vi "IMAQdx Read Memory2.vi"(8 "error in":errorcluster, 9 "Memory Size":u32, 10 "Offset":u64=4042262528 format="%.0x", 11 "Session In":T1) -> (0 "error out":errorcluster, 1 "Value":string, 3 "Session Out":T1)   [LabVIEW 2020, in "NI_Vision_Acquisition_Software.lvlib"]
doc: "Accesses registers on the camera and reads a string from the camera."
uses:
  NI_Vision_Acquisition_Software.lvlib
  IMAQdx.ctl
  niimaqdx.dll
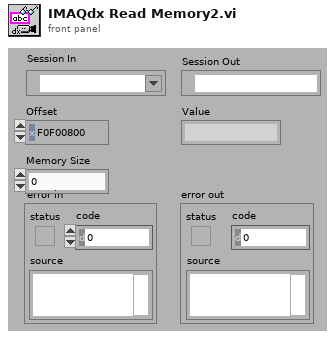
[diagram p1: front panel]
types:
  T1 = typedef "IMAQdx.ctl" = refnum<k21>
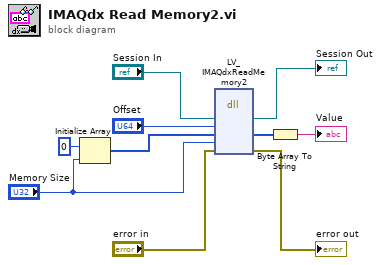
[diagram p0: block diagram]
diagram:
  n1 = Initialize Array(u8 0 ("element"), "Memory Size") -> (w3:u8[])
  n2 = dll-call lib="niimaqdx.dll" fn="LV_IMAQdxReadMemory2"("refNum"="Session In", "offset"="Offset", "array"=w3, "count"="Memory Size", "err"="error in") -> ("refNum"=→"Session Out":T1, "array"=w2:u8[], "err"=→"error out":errorcluster)  [unwired: 6 in, 2 out]
  n3 = Byte Array To String(unsigned byte array=w2) -> (string=→"Value":string)
